vi "SimulatedToArray.vi"(8 "Minimum Angle":i8=-90, 9 "Maximum Angle":i8=90, 10 "Number of Elements":u8=7, 11 "Degree":i8) -> (0 "Value Array":u16[](array[numeric]))   [LabVIEW 2013]
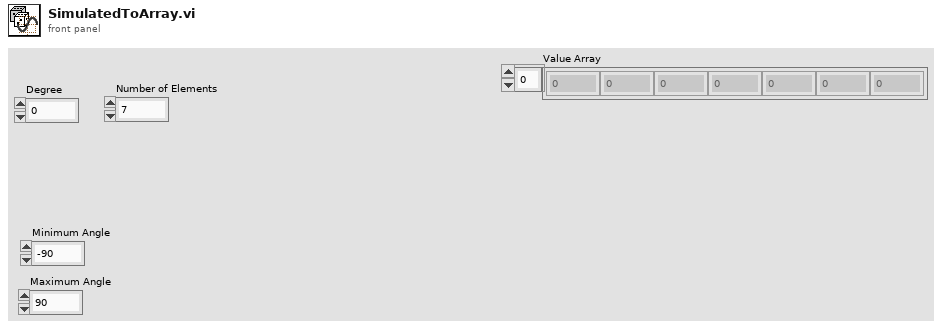
[diagram p1: front panel]
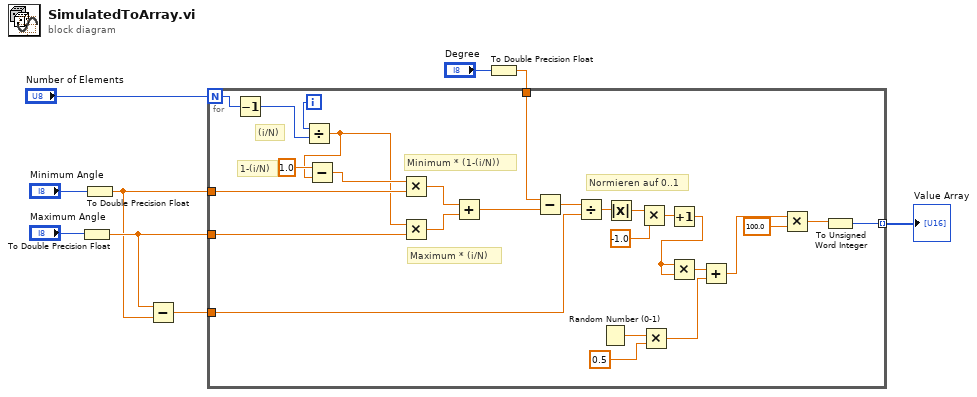
[diagram p0: block diagram]
diagram:
  n1 = To Double Precision Float(number="Maximum Angle") -> (double precision float=w3:dbl)
  n2 = To Double Precision Float(number="Minimum Angle") -> (double precision float=w2:dbl)
  n3 = Subtract(x=w3, y=w2) -> (x-y=w1:dbl)
  n4 = To Double Precision Float(number="Degree") -> (double precision float=w4:dbl)
  n5 = for {
    N: "Number of Elements" -> [w28]
    tunnel: w2 -> [w34]
    tunnel: w3 -> [w32]
    tunnel: [w10] -> w7 mode=indexing
    tunnel: w4 -> [w25]
    tunnel: w1 -> [w23]
    i -> [w29]
    # "Normieren auf 0..1"
    # "Maximum * (i/N)"
    # "Minimum * (1-(i/N))"
    # "(i/N)"
    # "1-(i/N)"
    n6 = Decrement(x=w28) -> (x-1=w27:i32)
    n7 = Divide(x=w29, y=w27) -> (x/y=w33:dbl)
    n8 = Subtract(x=1.0, y=w33) -> (x-y=w35:dbl)
    n9 = Multiply(x=w35, y=w34) -> (x*y=w31:dbl)
    n10 = Multiply(x=w33, y=w32) -> (x*y=w30:dbl)
    n11 = Add(x=w31, y=w30) -> (x+y=w26:dbl)
    n12 = Subtract(x=w25, y=w26) -> (x-y=w24:dbl)
    n13 = Divide(x=w24, y=w23) -> (x/y=w22:dbl)
    n14 = Random Number (0-1)() -> (number: 0 to 1=w16:dbl)
    n15 = Absolute Value(x=w22) -> (abs(x)=w21:dbl)
    n16 = Multiply(x=w21, y=-1.0) -> (x*y=w19:dbl)
    n17 = Multiply(x=w16, y=0.5) -> (x*y=w15:dbl)
    n18 = Increment(x=w19) -> (x+1=w18:dbl)
    n19 = Multiply(x=w18, y=w18) -> (x*y=w17:dbl)
    n20 = Add(x=w17, y=w15) -> (x+y=w13:dbl)
    n21 = Multiply(x=w13, y=100.0) -> (x*y=w11:dbl)
    n22 = To Unsigned Word Integer(number=w11) -> (unsigned 16bit integer=w10:u16)
  }
  "Value Array" <- w7
